vi "ResettableTimer.vi"(11 "Restart timer?":bool) -> (3 "Time since last reset":dbl)   [LabVIEW 2012]
doc: "This VI times how long it's been since the boolean was last triggered. After being triggered, the timer rezeros and then outputs the time since that triggering.\n\nEric Schneider, Jan. 2014"
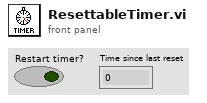
[diagram p1: front panel]
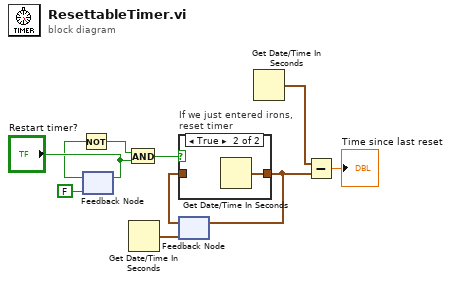
[diagram p0: block diagram]
diagram:
  n1 = feedback #1(FALSE ("InIrons?")) -> (w5:bool)
  n2 = Not(x=w5) -> (.not. x?=w8:bool)
  n3 = feedback-in #1("Restart timer?") -> ()
  n4 = And(x=w8, y="Restart timer?") -> (x .and. y?=w4:bool)
  n5 = Get Date/Time In Seconds() -> (seconds since 1Jan1904=w2:timestamp)
  n6 = feedback #2(w2) -> (w3:timestamp)
  n7 = case "If we just entered irons,\nreset timer" shown="True" w4 {
    tunnel: [w11 w12] -> w1
    tunnel: w3 -> [w11 _]
    frame False {
    }
    frame True {
      n8 = Get Date/Time In Seconds() -> (seconds since 1Jan1904=w12:timestamp)
    }
  }
  n9 = feedback-in #2(w1) -> ()
  n10 = Get Date/Time In Seconds() -> (seconds since 1Jan1904=w7:timestamp)
  n11 = Subtract(x=w7, y=w1) -> (x-y=→"Time since last reset":dbl)
